vi "Initialize multlist.vi"(10 "Type":enum16{"Volt", "Current"}(ring)=enum."Current") -> (2 "Item Names":string[][](array[string]))   [LabVIEW 2017]
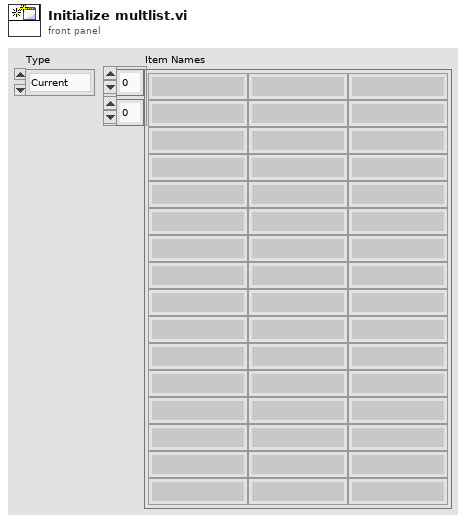
[diagram p1: front panel]
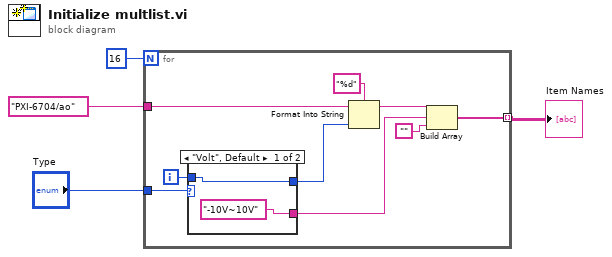
[diagram p0: block diagram]
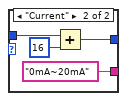
[diagram p2: hidden frame]
diagram:
  n1 = for {
    N: 16 -> [_]
    tunnel: "PXI-6704/ao" -> [w13]
    tunnel: "Type" -> [w11]
    tunnel: [w5] -> w1 mode=indexing
    i -> [w10]
    n2 = case shown="\"Volt\", Default" w11 {
      tunnel: w10 -> [w15 w19]
      tunnel: [w15 w17] -> w9
      tunnel: ["-10V~10V" "0mA~20mA"] -> w7
      frame "Volt", Default {
      }
      frame "Current" {
        n3 = Add(x=w19, y=16) -> (x+y=w17:i32)
      }
    }
    n4 = Format Into String(format string="%d", initial string=w13, w9) -> (resulting string=w8:string)  [unwired: 1 in, 1 out]
    n5 = Build Array(w8, w7, "") -> (w5:string[])
  }
  "Item Names" <- w1
